vi "Read AOinitialised.vi"(8 "error in (no error)":errorcluster, 11 "AO in":T1) -> (0 "error out":errorcluster, 2 "initialised":u8, 3 "AO out":T1)   [LabVIEW 2019, in "Inputs.lvlib"]
uses:
  Inputs.lvlib
  Ctl/AO.ctl
  Ctl/Parameter State.ctl
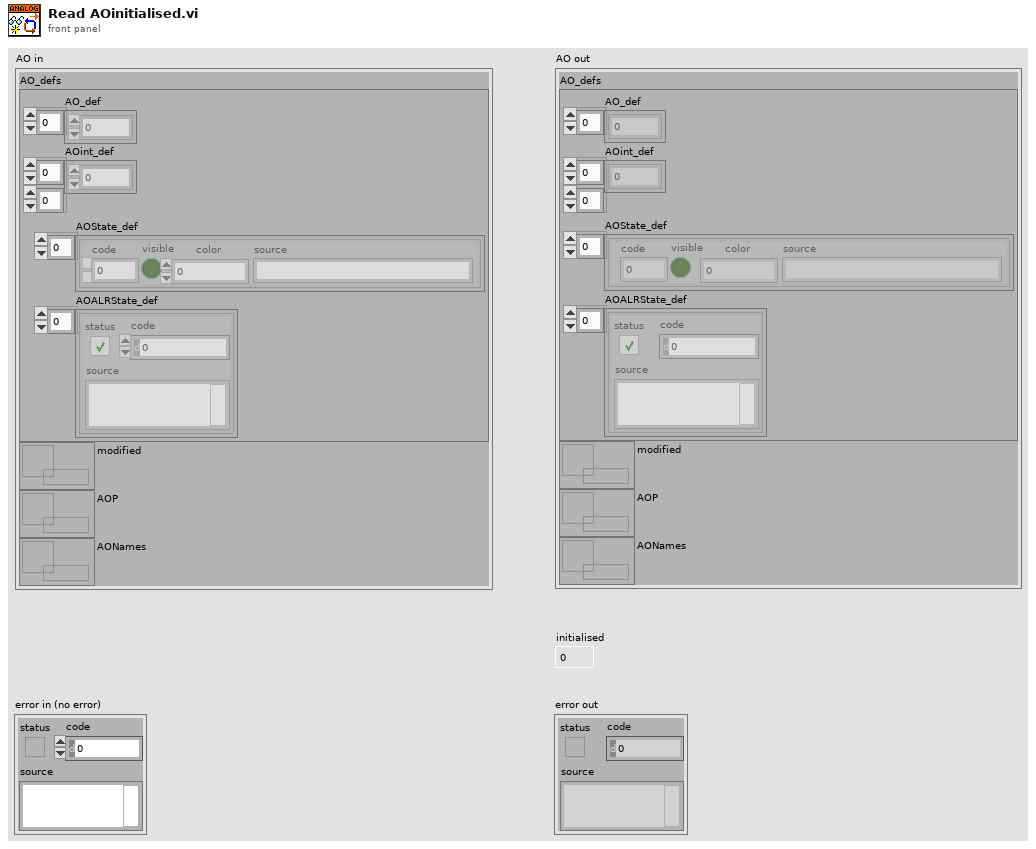
[diagram p1: front panel]
types:
  T1 = typedef "Inputs.lvlib/AO.ctl" = cluster{"AO_defs":cluster{"AO_def":dbl[], "AOint_def":u16[][], "AOState_def":T2[], "AOALRState_def":errorcluster[]}, "modified":refnum<data-value>, "AOP":refnum<data-value>, "AONames":refnum<data-value>}
  T2 = typedef "Inputs.lvlib/Parameter State.ctl" = cluster{"code":i32, "visible":bool, "color":u32, "source":string}
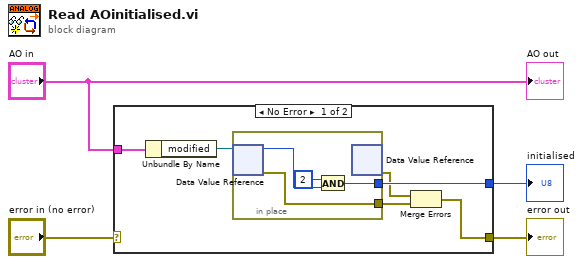
[diagram p0: block diagram]
diagram:
  n1 = case shown="No Error" "error in (no error)" {
    selector: "error in (no error)" -> [_ w15]
    tunnel: [w6 w15] -> w3
    tunnel: "AO in" -> [w5 _]
    tunnel: [w9 _] -> w4
    frame No Error {
      n2 = Unbundle By Name(w5) -> ("modified"=w10:refnum<data-value>)
      n3 = in-place {
        in-place-border: [w14] -> w8
        in-place-border: [w12] -> w9
        n4 = in-place-dvr #1(w10) -> (w13:u8, w14:errorcluster)
        n5 = And(x=u8 2, y=w13) -> (x .and. y?=w12:u8)
        n6 = in-place-dvr #1() -> (w7:errorcluster)  [unwired: 1 in, 1 out]
      }
      n7 = Merge Errors(w7, w8) -> (w6:errorcluster)
    }
    frame Error {
    }
  }
  "error out" <- w3
  "initialised" <- w4
  "AO out" <- "AO in"
